vi "Sub_Build_MQTT_PubPayload_String.vi"(8 "error in (no error)":errorcluster, 10 "String to be encoded":string="MQIsdp") -> (0 "error out":errorcluster, 2 "UTF8 Byte Array":u8[](array[numeric]) format="%x")   [LabVIEW 2019, in "MQTT_Functions.lvlib"]
uses:
  MQTT_Functions.lvlib
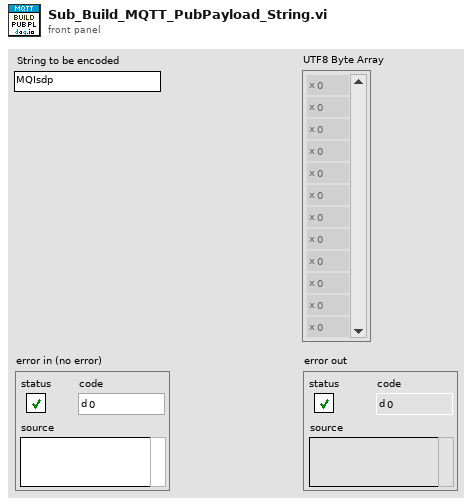
[diagram p1: front panel]
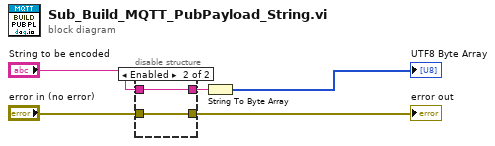
[diagram p0: block diagram]
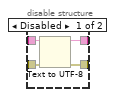
[diagram p2: hidden frame]
diagram:
  n1 = disable-structure shown="Enabled" {
    disable-tunnel: "String to be encoded" -> [w9 w11]
    disable-tunnel: "error in (no error)" -> [w8 w10]
    disable-tunnel: [w7 w11] -> w3
    disable-tunnel: [w6 w10] -> w2
    frame Disabled {
      n2 = Text to UTF-8(8:w8, 11:w9) -> (0:w6:errorcluster, 3:w7:string)  [unwired: 1 in]
    }
    frame Enabled {
    }
  }
  "error out" <- w2
  n3 = String To Byte Array(string=w3) -> (unsigned byte array=→"UTF8 Byte Array":u8[])
